vi "Property Tree_Build Tree.vi"(6 "Close Items":bool, 7 "Action":T4, 8 "error in":errorcluster, 9 "Filter":T1, 10 "Properties for Tree":T3(array[cluster]), 11 "Tree Ref":refnum<vi>) -> (0 "error out":errorcluster, 1 "Displayed Items":string[](array[string]), 3 "Tree Ref Out":refnum<vi>, 4 "exe time (ms)":u32)   [LabVIEW 2023]
doc: "Take a cluster reference and build a tree of all items in cluster. Set tags of items as \"[row number] item name\" so all tags are unique. Set glyph of its to indicate data type. Set selection color to gray and font size to 18pt.\n\nThis VI mainly deals with row-level properties."
uses:
  controls/action enum.ctl
panel:
  out "Tree Arr":T2(array[cluster])
  in  "Tree":string[](tree)
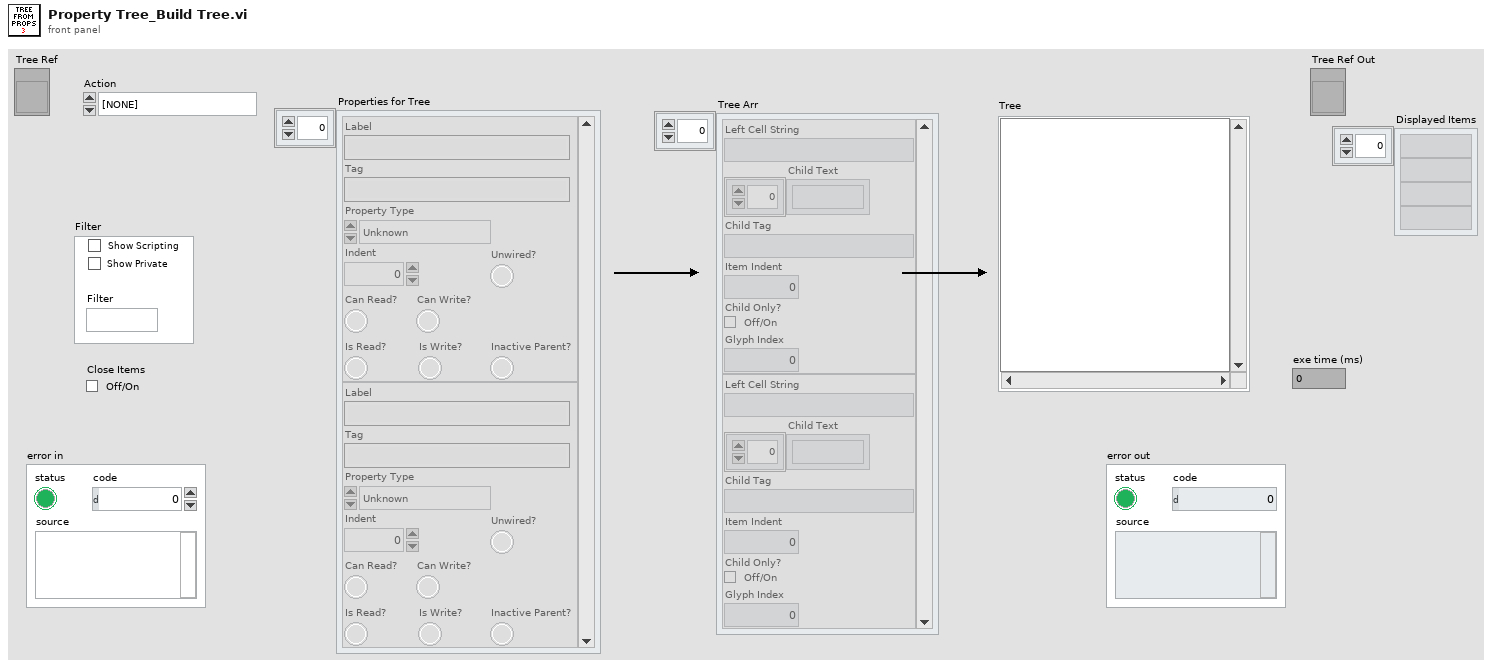
[diagram p1: front panel]
types:
  T1 = cluster{"Show":cluster{"Show Scripting":bool, "Show Private":bool}, "Filter":string}
  T2 = cluster{"Left Cell String":string, "Child Text":string[], "Child Tag":string, "Item Indent":i32, "Child Only?":bool, "Glyph Index":i32}[]
  T3 = cluster{"Label":string, "Tag":string, "Property Type":enum16{"Unknown", "Base", "Scripting", "Private", "Deprecated", "None", "Divider"}, "Indent":u16, "Can Read?":bool, "Can Write?":bool, "Is Read?":bool, "Is Write?":bool, "Inactive Parent?":bool, "Unwired?":bool}[]
  T4 = typedef "action enum.ctl" = enum16{"[NONE]", "Wire Bundle", "Wire Unbundle", "Terminal Unbundle", "Terminal Bundle", "Bundler Move Up", "Bundler Move Down", "Bundler Insert", "Bundler Remove", "Bundler Remove Unwired", "Bundler Rearrange", "In Place Insert", "In Place Remove", "In Place Remove Unwired", "In Place Rearrange", "Wire Properties", "Wire Method", "Terminal Properties", "Terminal Method", "Property Move Up", "Property Move Down", "Properties Insert", "Properties Remove", "Properties Remove Unwired", "Properties Rearrange", "Method Change", "Class for Constant", "Class For Control", "Class For Node", "Class Name to Clipboard"}
  T5 = enum16{"Unknown", "Base", "Scripting", "Private", "Deprecated", "None", "Divider"}
  T6 = cluster{"Label":string, "Tag":string, "Property Type":enum16{"Unknown", "Base", "Scripting", "Private", "Deprecated", "None", "Divider"}, "Indent":u16, "Can Read?":bool, "Can Write?":bool, "Is Read?":bool, "Is Write?":bool, "Inactive Parent?":bool, "Unwired?":bool}
  T7 = cluster{"Show Scripting":bool, "Show Private":bool}
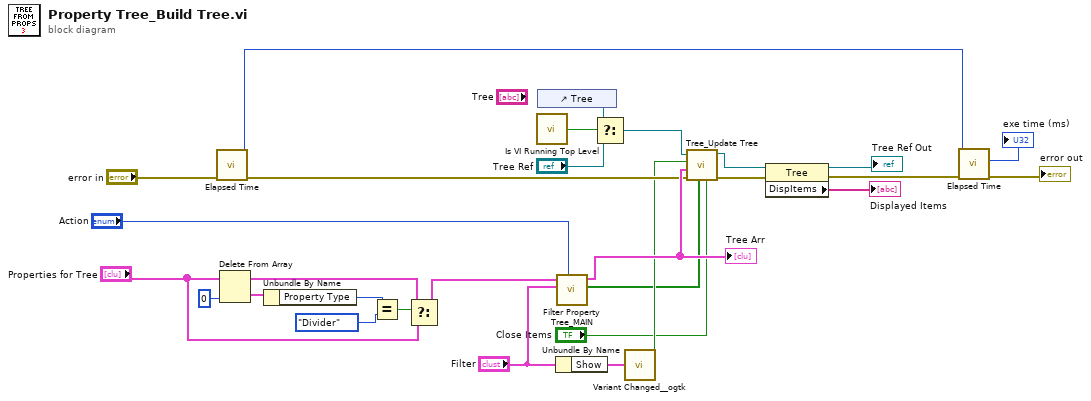
[diagram p0: block diagram]
diagram:
  n1 = call "Elapsed Time.vi"("error in"="error in") -> ("error out"=w15:errorcluster, "millisecond timer value"=w23:u32)  [unwired: 7 in, 2 out]
  n2 = Delete From Array(array="Properties for Tree", index=0) -> (deleted portion=w5:T6, array with subset deleted=w1:T3)  [unwired: 1 in]
  n3 = Unbundle By Name(w5) -> ("Property Type"=w4:T5)
  n4 = Equal?(x=w4, y=T5."Divider" ("Property Type")) -> (x = y?=w2:bool)
  n5 = Select(t=w1, s=w2, f="Properties for Tree") -> (s? t:f=w17:T3)
  n6 = call "Is VI Running Top Level.vi"() -> ("Top Level?"=w29:bool)  [unwired: 5 in]
  n7 = control-ref of="Tree"() -> (w27:refnum<vi>)
  n8 = Unbundle By Name("Filter") -> ("Show"=w11:T7)
  n9 = call "Filter Property Tree_MAIN.vi"("Action"="Action", "Filter"="Filter", "Properties for Tree In"=w17) -> ("Disabled?"=w8:bool[], "Tree Arr"=w22:T2)  [unwired: 7 in]
  "Tree Arr" <- w22
  n10 = Select(t=w27, s=w29, f="Tree Ref") -> (s? t:f=w16:refnum<vi>)
  n11 = call <userlib>:"Variant Changed__ogtk.vi"("Variant"=w11) -> ("Changed"=w10:bool)
  n12 = call "Tree_Update Tree.vi"("Close Items"="Close Items", "Disabled?"=w8, "error in"=w15, "New Items"=w22, "Show Changed"=w10, "TreeControl in"=w16) -> ("error out"=w13:errorcluster, "TreeControl out"=w14:refnum<vi>)  [unwired: 4 in]
  n13 = property class="Tree"(reference=w14, error in=w13) -> (reference out=→"Tree Ref Out":refnum<vi>, error out=w19:errorcluster, "DispItems"=→"Displayed Items":string[])
  n14 = call "Elapsed Time.vi"("error in"=w19, "past time"=w23) -> ("error out"=→"error out":errorcluster, "exe time (ms)"=→"exe time (ms)":u32)  [unwired: 6 in, 2 out]
